vi "dataBuffer.vi"(6 "command":T2=enum."read recent", 8 "error in (no error)":errorcluster, 10 "max array size":u16=5000 min=1, 11 "averaged data":T1) -> (0 "error out":errorcluster, 1 "recent time":timestamp, 2 "scans":i32, 3 "recent data":dbl[](array[numeric]), 5 "misc graph":cluster{timestamp[], dbl[]}[](graph), 7 "turbidity":cluster{timestamp[], dbl[]}[](graph))   [LabVIEW 2015]
uses:
  Sensor buffer command.ctl
  data array with time.ctl
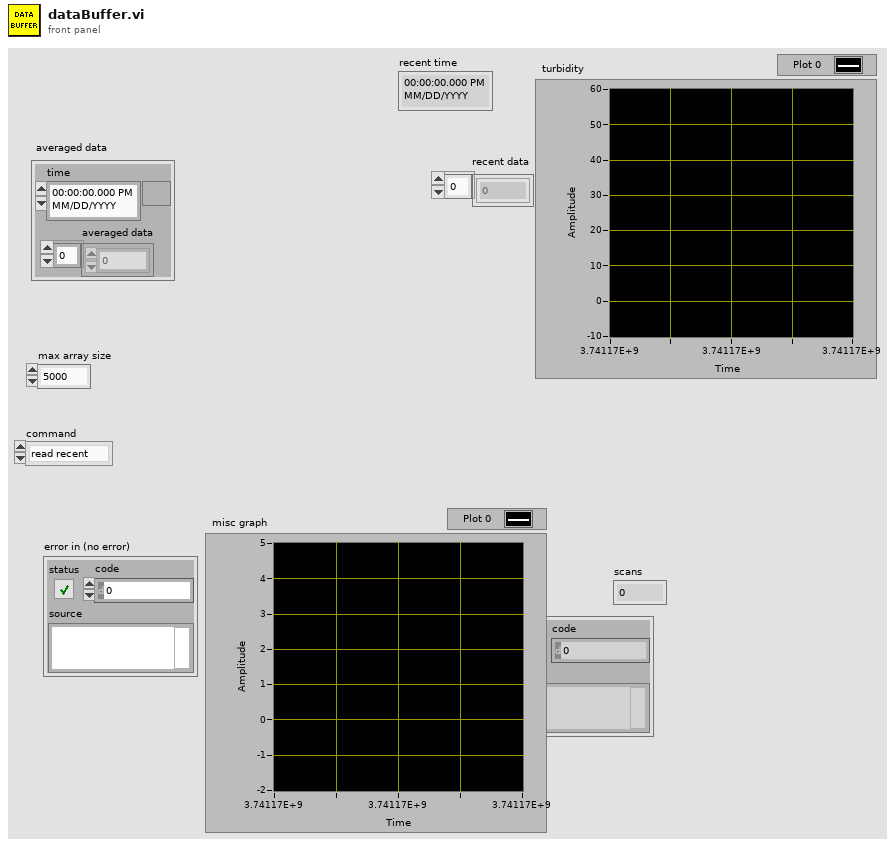
[diagram p1: front panel]
types:
  T1 = typedef "data array with time.ctl" = cluster{"time":timestamp, "averaged data":dbl[]}
  T2 = typedef "Sensor buffer command.ctl" = enum16{"set buffer size", "write", "refill buffer", "read recent", "read all", "clear"}
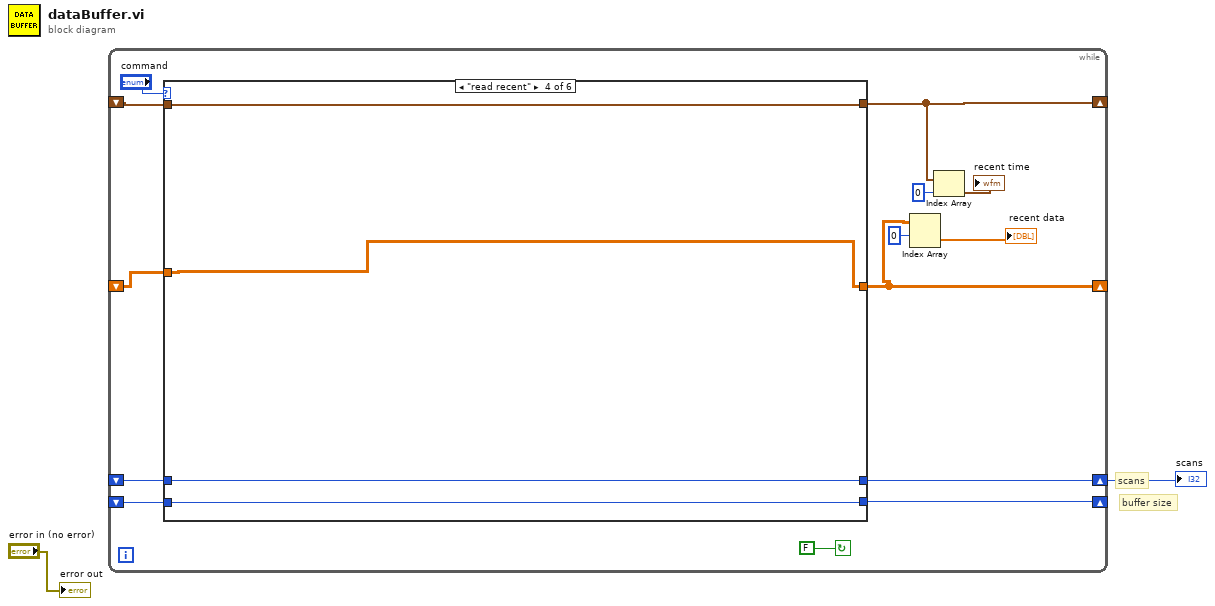
[diagram p0: block diagram]
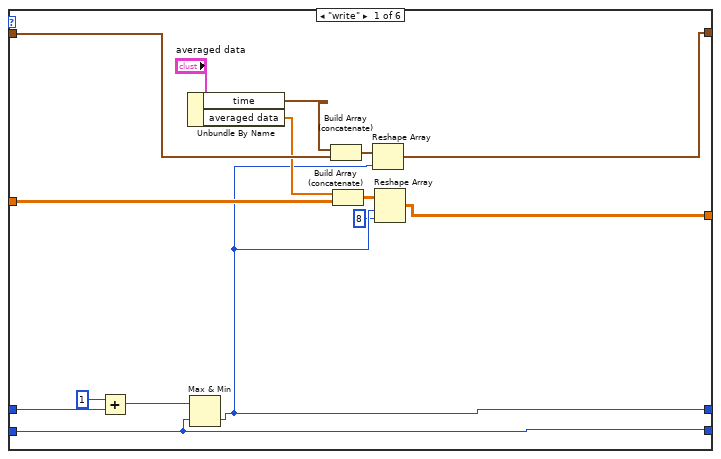
[diagram p2: hidden frame]
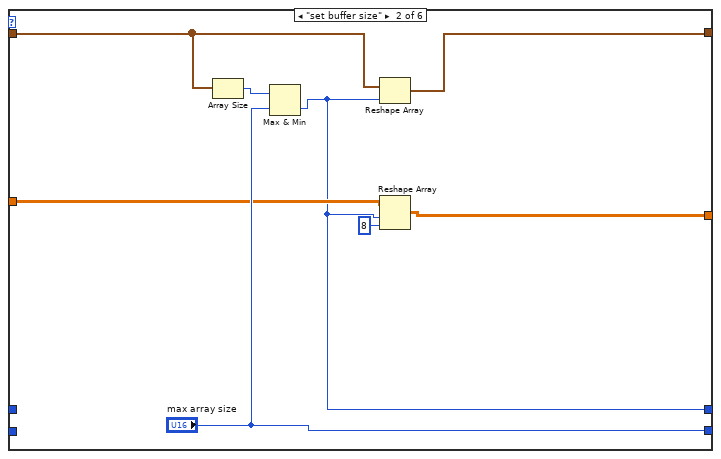
[diagram p3: hidden frame]
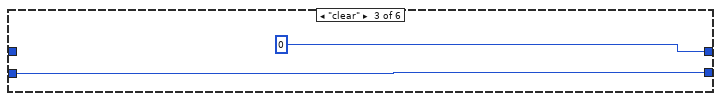
[diagram p4: hidden frame]
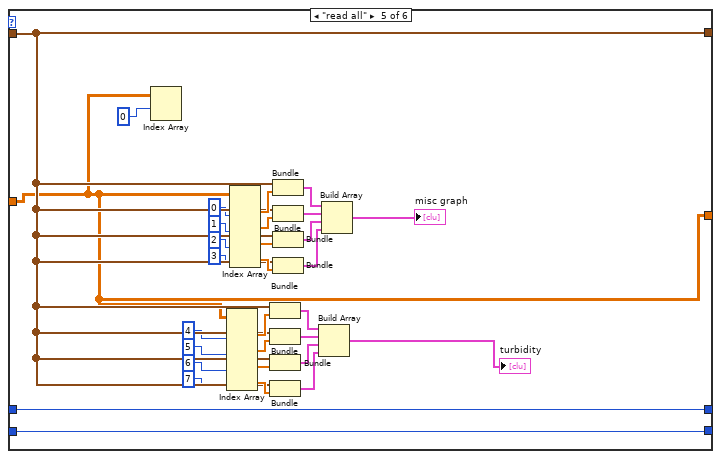
[diagram p5: hidden frame]
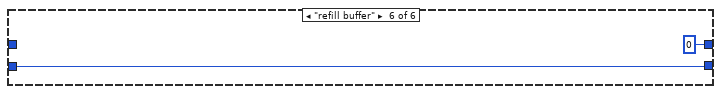
[diagram p6: hidden frame]
diagram:
  # "buffer size"
  # "scans"
  n1 = while {
    shift-right: [w3] -> _
    shift-left: _ -> [w15]
    shift-right: [w14] -> _
    shift-left: _ -> [w13]
    shift-right: [w10] -> w1
    shift-left: _ -> [w11]
    shift-right: [w6] -> _
    shift-left: _ -> [w9]
    stop <- FALSE continue-if-true
    n2 = case shown="\"read recent\"" "command" {
      tunnel: [w28 w39 _ w43 w56 _] -> w3
      tunnel: w15 -> [w30 w38 _ w43 w56 _]
      tunnel: [w26 "max array size" w41 w45 w76 w78] -> w14
      tunnel: w13 -> [w26 _ w41 w45 w76 w78]
      tunnel: w11 -> [w29 _ _ w44 w75 _]
      tunnel: [w18 w33 0 w44 w75 0] -> w10
      tunnel: [w20 w34 _ w42 w47 _] -> w6
      tunnel: w9 -> [w19 w35 _ w42 w47 _]
      frame "write" {
        n3 = Add(x=1, y=w29) -> (x+y=w25:i32)
        n4 = Unbundle By Name("averaged data") -> ("time"=w23:timestamp, "averaged data"=w21:dbl[])
        n5 = Max & Min(x=w25, y=w26) -> (min(x,y)=w18:i32)  [unwired: 1 out]
        n6 = Build Array (concatenate)(w23, w30) -> (w27:timestamp[])
        n7 = Build Array (concatenate)(w21, w19) -> (w22:dbl[][])
        n8 = Reshape Array(w27, w18) -> (w28:timestamp[])
        n9 = Reshape Array(w22, w18, 8 ("dimension size")) -> (w20:dbl[][])
      }
      frame "set buffer size" {
        n10 = Array Size(array=w38) -> (size(s)=w37:i32)
        n11 = Max & Min(x=w37, y="max array size") -> (min(x,y)=w33:i32)  [unwired: 1 out]
        n12 = Reshape Array(w38, w33) -> (w39:timestamp[])
        n13 = Reshape Array(w35, w33, 8 ("dimension size")) -> (w34:dbl[][])
      }
      frame "clear" {
      }
      frame "read recent" {
      }
      frame "read all" {
        n14 = Index Array(array=w47, index (row)=0) -> ()  [unwired: 1 in, 1 out]
        n15 = Index Array(array=w47, index (col) #1=4 ("index (row)"), index (col) #2=5 ("index (row)"), index (col) #3=6 ("index (row)"), index (col) #4=7 ("index (row)")) -> (element #1=w58:dbl[], element #2=w59:dbl[], element #3=w60:dbl[], element #4=w61:dbl[])  [unwired: 4 in]
        n16 = Index Array(array=w47, index (col) #1=0 ("index (row)"), index (col) #2=1 ("index (row)"), index (col) #3=2 ("index (row)"), index (col) #4=3 ("index (row)")) -> (element #1=w74:dbl[], element #2=w73:dbl[], element #3=w72:dbl[], element #4=w71:dbl[])  [unwired: 4 in]
        n17 = Bundle(w56, w58) -> (w62:cluster{timestamp[], dbl[]})  [unwired: 1 in]
        n18 = Bundle(w56, w59) -> (w63:cluster{timestamp[], dbl[]})  [unwired: 1 in]
        n19 = Bundle(w56, w60) -> (w64:cluster{timestamp[], dbl[]})  [unwired: 1 in]
        n20 = Bundle(w56, w61) -> (w65:cluster{timestamp[], dbl[]})  [unwired: 1 in]
        n21 = Bundle(w56, w74) -> (w70:cluster{timestamp[], dbl[]})  [unwired: 1 in]
        n22 = Bundle(w56, w73) -> (w69:cluster{timestamp[], dbl[]})  [unwired: 1 in]
        n23 = Bundle(w56, w72) -> (w67:cluster{timestamp[], dbl[]})  [unwired: 1 in]
        n24 = Bundle(w56, w71) -> (w66:cluster{timestamp[], dbl[]})  [unwired: 1 in]
        n25 = Build Array(w62, w63, w64, w65) -> (→"turbidity":cluster{timestamp[], dbl[]}[])
        n26 = Build Array(w70, w69, w67, w66) -> (→"misc graph":cluster{timestamp[], dbl[]}[])
      }
      frame "refill buffer" {
      }
    }
    n27 = Index Array(array=w6, index (row)=0 ("index")) -> (element=→"recent data":dbl[])  [unwired: 1 in]
    n28 = Index Array(array=w3, index=0) -> (element=→"recent time":timestamp)
  }
  "scans" <- w1
  "error out" <- "error in (no error)"
